vi "to string.vi"(8 "error in":errorcluster, 11 "module configuration in":refnum<class "fixed channel tag bus module configuration.lvclass">) -> (0 "error out":errorcluster, 1 "data":string, 2 "version":string, 3 "module configuration out":refnum<class "fixed channel tag bus module configuration.lvclass">)   [LabVIEW 2013, in "fixed channel tag bus module configuration.lvclass"]
doc: "Provides an interface for saving a module configuration to a file or other serialized data source. It is recommended that all children of this class store data in two sets--data required for its own initialization, and any data required for parent initialization--and that each implementation uses the <b>Call Parent Method</b> primitive to serialize parent information.\nNI Tag Bus Module Framework 1.0.3.43\nNI Systems Engineering"
uses:
  fixed channel tag bus module configuration.lvclass
  <vilib>/NI/Tag Bus Module Framework/module configuration/TBM module configuration.lvclass
  fixed channel tag bus module configuration.lvclass/fixed channel tag bus module configuration.ctl
  <vilib>/NI/Tag Bus Module Framework/channel/TBM channel.lvclass
  <vilib>/NI/Tag Bus Module Framework/root configuration/TBM configuration.lvclass
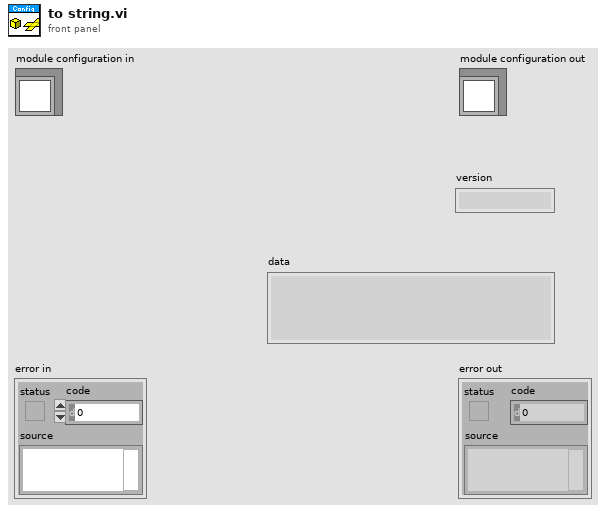
[diagram p1: front panel]
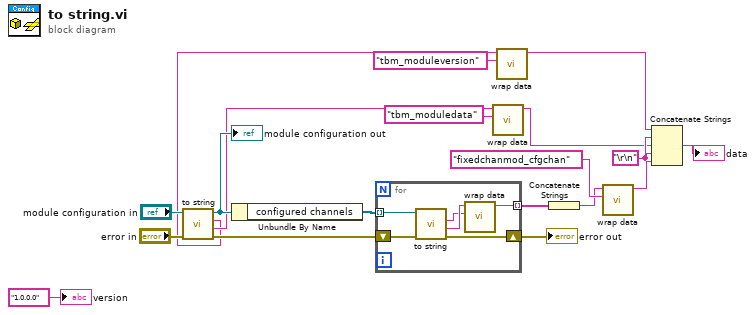
[diagram p0: block diagram]
diagram:
  w7 = "\r\n"
  n1 = call-parent "to string.vi"("error in"="error in", "module configuration in"="module configuration in") -> ("error out"=w15:errorcluster, "data"=w4:string, "version"=w3:string, "module configuration out"=w17:refnum<class "fixed channel tag bus module configuration.lvclass">)  [unwired: 6 in]
  "module configuration out" <- w17
  n2 = Unbundle By Name(w17) -> ("configured channels"=w13:refnum<class "TBM channel.lvclass">[])
  n3 = for {
    tunnel: w13 -> [w25] mode=indexing
    shift-right: [w21] -> w14
    shift-left: w15 -> [w22]
    tunnel: [w20] -> w9 mode=indexing
    n4 = call-dynamic "to string.vi"("error in"=w22, "channel in"=w25) -> ("error out"=w21:errorcluster, "channel data"=w24:string, "identifier"=w23:string)  [unwired: 6 in, 1 out]
    n5 = call <vilib>:"wrap data.vi"("identifier"=w23, "data to wrap"=w24) -> ("wrapped data"=w20:string)  [unwired: 9 in]
  }
  "error out" <- w14
  n6 = call <vilib>:"wrap data.vi"("identifier"="tbm_moduledata", "data to wrap"=w4) -> ("wrapped data"=w6:string)  [unwired: 9 in]
  n7 = call <vilib>:"wrap data.vi"("identifier"="tbm_moduleversion", "data to wrap"=w3) -> ("wrapped data"=w5:string)  [unwired: 9 in]
  n8 = Concatenate Strings(w9) -> (w8:string)
  n9 = call <vilib>:"wrap data.vi"("identifier"="fixedchanmod_cfgchan", "data to wrap"=w8) -> ("wrapped data"=w12:string)  [unwired: 9 in]
  n10 = Concatenate Strings(w5, w7, w6, w7, w12) -> (→"data":string)
  "version" <- "1.0.0.0" ("version")
